vi "tearDown.vi"(8 "error in (no error)":errorcluster, 11 "reference in":refnum<class "Test Network Stream Initiator Connect.lvclass">) -> (0 "error out":errorcluster, 3 "reference out":refnum<class "Test Network Stream Initiator Connect.lvclass">)   [LabVIEW 2020, in "Test Network Stream Initiator Connect.lvclass"]
doc: "tearDown runs after the test method has completed. Use this method to clean up any operations or references that were opened by setUp or the test method. Unit tests should be independent of other unit tests so this VI should ensure that the next test can run in a 'clean' test environment."
uses:
  Test Network Stream Initiator Connect.lvclass
  Source/Protocols/Network Stream Strategy/Network Stream Initiator/Network Stream Initiator.lvclass
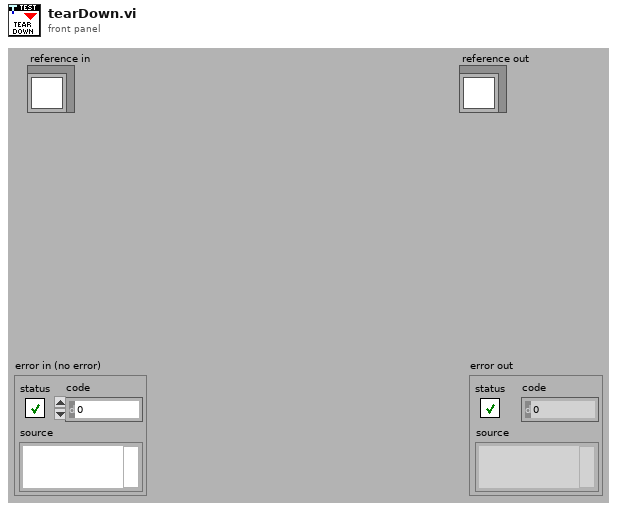
[diagram p1: front panel]
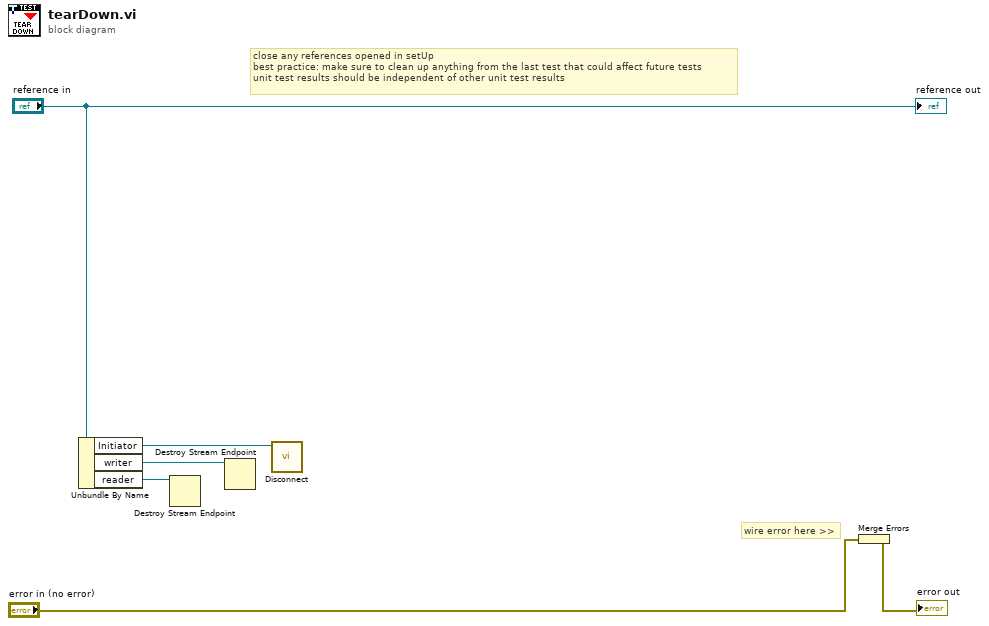
[diagram p0: block diagram]
diagram:
  # "wire error here >>"
  # "close any references opened in setUp\nbest practice: make sure to clean up anything from the last test that could affect future tests\nunit test results should be independent of other unit test results"
  n1 = Unbundle By Name("reference in") -> ("Initiator"=w3:refnum<class "Network Stream Initiator.lvclass">, "writer"=w2:refnum<k21>, "reader"=w1:refnum<k21>)
  n2 = Destroy Stream Endpoint(11:w1) -> ()  [unwired: 1 in, 1 out]
  n3 = Destroy Stream Endpoint(11:w2) -> ()  [unwired: 1 in, 1 out]
  n4 = call-dynamic "Disconnect.vi"("Network Stream in"=w3) -> ()  [unwired: 9 in, 2 out]
  n5 = Merge Errors("error in (no error)") -> (→"error out":errorcluster)
  "reference out" <- "reference in"
